vi "Channels to Define.vi"(8 "error in (no error)":errorcluster, 11 "JSON Routing Channel Template in":refnum<class "JSON Routing Channel Template.lvclass">) -> (0 "error out":errorcluster, 2 "Channels":string[](array[string]), 3 "JSON Routing Channel Template out":refnum<class "JSON Routing Channel Template.lvclass">)   [LabVIEW 2020, in "Routing Templates.lvlib" / "JSON Routing Channel Template.lvclass"]
uses:
  JSON Routing Channel Template.lvclass
  JSON Routing Channel Template.lvclass/JSON Routing Channel Template.ctl
  Abstract Routing Channel Template/Abstract Routing Channel Template.lvclass
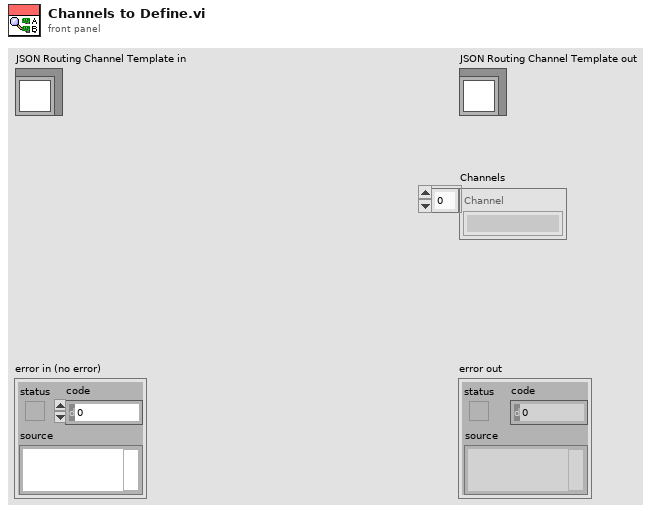
[diagram p1: front panel]
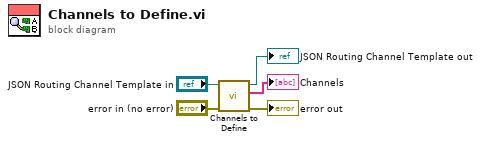
[diagram p0: block diagram]
diagram:
  n1 = call-parent "Channels to Define.vi"("error in (no error)"="error in (no error)", "Abstract Routing Channel Template in"="JSON Routing Channel Template in") -> ("error out"=→"error out":errorcluster, "Channels"=→"Channels":string[], "Abstract Routing Channel Template out"=→"JSON Routing Channel Template out":refnum<class "JSON Routing Channel Template.lvclass">)  [unwired: 7 in]
